vi "select spots Sub_1.vi"(0 "Ring Refnum":refnum<vi>, 1 "Ring Refnum 2":refnum<vi>, 2 "Ring Refnum 3":refnum<vi>, 3 "Ring Refnum 4":refnum<vi>, 4 "file (use dialog)":path) -> (5 "names":string[](array[string]), 6 "Array":dbl[][](array[numeric]))   [LabVIEW 2009]
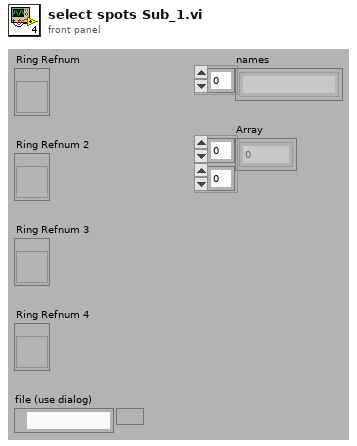
[diagram p1: front panel]
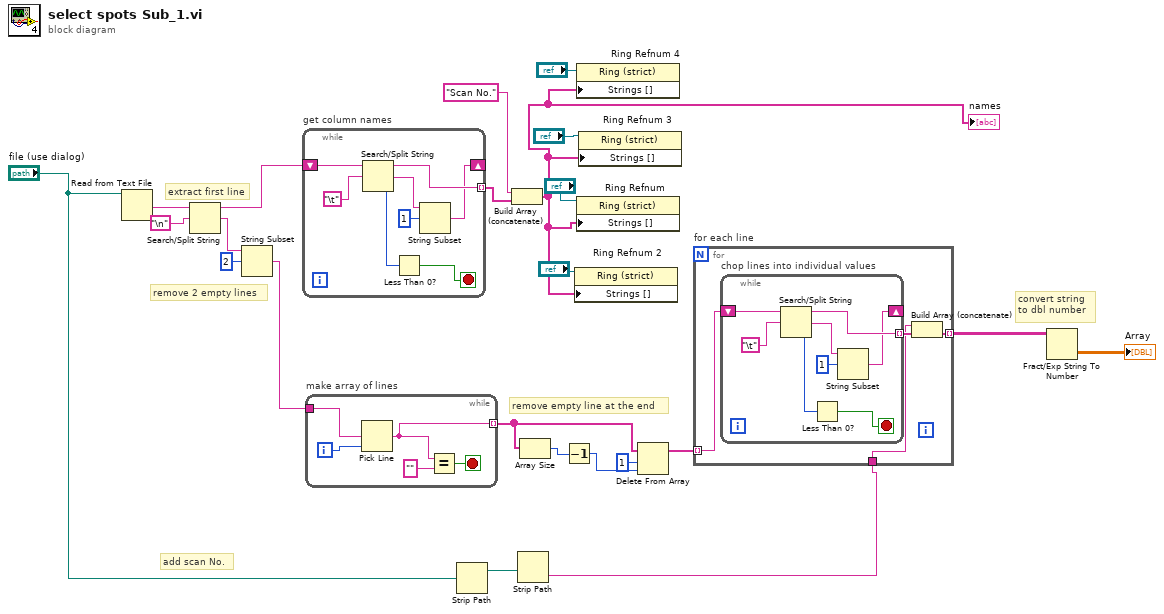
[diagram p0: block diagram]
diagram:
  # "add scan No."
  # "convert string \nto dbl number"
  # "extract first line"
  # "remove empty line at the end"
  # "remove 2 empty lines"
  n1 = Read from Text File(file (use dialog)="file (use dialog)") -> (text=w12:string)  [unwired: 3 in, 3 out]
  n2 = Search/Split String(string=w12, search string/char (-)="\n") -> (substring before match=w16:string, match + rest of string=w14:string)  [unwired: 1 in, 1 out]
  n3 = String Subset(string=w14, offset (0)=2) -> (substring=w23:string)  [unwired: 1 in]
  n4 = while "get column names" {
    tunnel: [w29] -> w6 mode=indexing
    shift-right: [w26] -> _
    shift-left: w16 -> [w31]
    stop <- w24 stop-if-true
    n5 = Search/Split String(string=w31, search string/char (-)="\t") -> (substring before match=w29:string, match + rest of string=w28:string, offset of match=w25:i32)  [unwired: 1 in]
    n6 = Less Than 0?(x=w25) -> (x < 0?=w24:bool)
    n7 = String Subset(string=w28, offset (0)=1) -> (substring=w26:string)  [unwired: 1 in]
  }
  n8 = while "make array of lines" {
    tunnel: w23 -> [w36]
    tunnel: [w33] -> w18 mode=indexing
    i -> [w32]
    stop <- w34 stop-if-true
    n9 = Pick Line(multi-line string=w36, line index=w32) -> (output string=w33:string)  [unwired: 1 in]
    n10 = Equal?(x=w33, y="") -> (x = y?=w34:bool)
  }
  n11 = Strip Path(path="file (use dialog)") -> (stripped path=w2:path)  [unwired: 1 out]
  n12 = Build Array (concatenate)("Scan No.", w6) -> (w4:string[])
  "names" <- w4
  n13 = Strip Path(path=w2) -> (name=w1:string)  [unwired: 1 out]
  n14 = Array Size(array=w18) -> (size(s)=w17:i32)
  n15 = Decrement(x=w17) -> (x-1=w19:i32)
  n16 = property on="Property Node" class="Ring (strict)"(reference="Ring Refnum 2", "Strings []"=w4) -> ()  [unwired: 1 in, 2 out]
  n17 = property on="Property Node" class="Ring (strict)"(reference="Ring Refnum 4", "Strings []"=w4) -> ()  [unwired: 1 in, 2 out]
  n18 = property on="Property Node" class="Ring (strict)"(reference="Ring Refnum", "Strings []"=w4) -> ()  [unwired: 1 in, 2 out]
  n19 = property on="Property Node" class="Ring (strict)"(reference="Ring Refnum 3", "Strings []"=w4) -> ()  [unwired: 1 in, 2 out]
  n20 = Delete From Array(array=w18, length=1, index=w19) -> (array with subset deleted=w21:string[])  [unwired: 1 out]
  n21 = for "for each line" {
    tunnel: w21 -> [w40] mode=indexing
    tunnel: [w39] -> w22 mode=indexing
    tunnel: w1 -> [w37]
    n22 = while "chop lines into individual values" {
      tunnel: [w46] -> w38 mode=indexing
      shift-right: [w43] -> _
      shift-left: w40 -> [w48]
      stop <- w41 stop-if-true
      n23 = Search/Split String(string=w48, search string/char (-)="\t") -> (substring before match=w46:string, match + rest of string=w45:string, offset of match=w42:i32)  [unwired: 1 in]
      n24 = Less Than 0?(x=w42) -> (x < 0?=w41:bool)
      n25 = String Subset(string=w45, offset (0)=1) -> (substring=w43:string)  [unwired: 1 in]
    }
    n26 = Build Array (concatenate)(w37, w38) -> (w39:string[])
  }
  n27 = Fract/Exp String To Number(string=w22) -> (number=→"Array":dbl[][])  [unwired: 3 in, 1 out]
